vi "SR1.get Number of Lines.vi"(0 "i ref in":refnum<vi>, 5 "error in (no error)":errorcluster) -> (14 "i ref out":refnum<vi>, 16 "NofLines":i32, 19 "error out":errorcluster)   [LabVIEW 2014, in "SR1.lvlib"]
doc: "reads the number of FFT lines from the device"
uses:
  SR1.lvlib
  CSlibraries/UtilityLib/UtilityLib.valueStatus.ctl
  CS_Core/CSApplicationBaseClasses/NABase/NABase.directionType.ctl
  CS_Core/CSApplicationBaseClasses/NABase/NABase.serviceType.ctl
  CS_Core/CSSystem/CoreDefs/CoreDefs.error_type.ctl
  CS_Core/CSSystem/CoreLib/CoreLib.lvlib
  CSlibraries/UtilityLib/UtilityLib.lvlib
  CS_Core/CSApplicationBaseClasses/NABase/NABase.lvlib
  instr.lib/Stanford Research SR1/Stanford Research SR1.lvlib
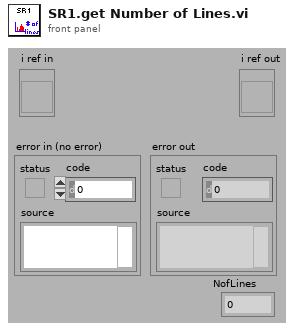
[diagram p1: front panel]
types:
  T1 = typedef "NABase.lvlib/NABase.serviceType.ctl" = enum16{"StartFreq", "NofLines", "FreqSpan", "status", "triggerLevel", "triggerSlope", "TimeRecDur", "NofStoredData"}
  T2 = typedef "NABase.lvlib/NABase.directionType.ctl" = enum16{"unknown", "update actual value", "update nominal value", "update both"}
  T3 = typedef "UtilityLib.lvlib/UtilityLib.valueStatus.ctl" = enum16{"no info available", "stand by/off", "on", "warning", "alarm/malfunction", "not implemented", "user action required", "important information", "system default", "control default", "indicator default", "button default"}
  T4 = typedef "CoreDefs.error_type.ctl" = enum16{"no error", "can't load process", "can't unload process", "process does not exist", "can't install process", "can't remove process", "unknown function", "time out", "can't execute function", "duplicate queue name", "super not found", "caller queue invalid", "can't ping process", "unknown error", "VISA Error", "VISA timeout", "GPIB timeout", "GPIB error", "communication error", "data type mismatch", "can't read data from OPC server", "can't write data to OPC server", "OET error", "function not implemented", "process already exists", "invalid Shared Variable name", "error writing Shared Variable", "error reading Shared Variable", "invalid client name", "corrupt database", "unknown class", "call not authorized", "parameter out of range", "OET timeout: can't get data to modify", "invalid queue name", "requested operation incompatible with current state", "event undefined", "event disabled", "state undefined", "caller is not a friend", "EventBuilder: bad eventID", "EventBuilder: no DAQ devices", "a thread must not stop itself", "UNUSED ELEMENT4", "DiscArchiver: eventData incomplete", "DiscArchiver: eventData does not belong to run", "DiscArchiver: can't open file", "DiscArchiver: can't write to file", "DiscArchiver: available disc space low", "can't acquire semaphore", "error reading data from database", "notifier object is not existing", "can't register process", "can't unregister process", "illegal event type", "object disabled", "object already exists", "can't change state", "Instrument not found", "no connection to remote node", "invalid reference", "N/A", "UNUSED ELEMENT 1", "element not found", "illegal TCP/IP connection detected", "object does not exist", "invalid access ID", "unknown CS system", "invalid privilige", "unsupported data type", "unsupported server type", "IO server already exists", "Shared Variable already exists"}
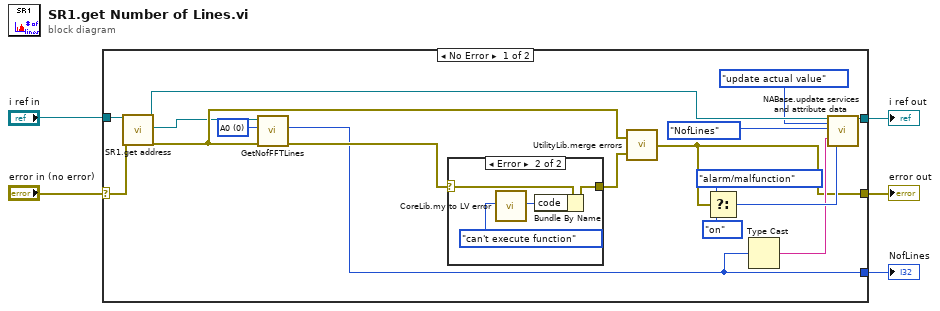
[diagram p0: block diagram]
diagram:
  n1 = case shown="No Error" "error in (no error)" {
    selector: "error in (no error)" -> [w20 w29]
    tunnel: "i ref in" -> [w22 w28]
    tunnel: [w13 w29] -> w4
    tunnel: [w14 w28] -> w3
    tunnel: [w6 _] -> w2
    frame No Error {
      w9 = 0 items=["A0", "A1"] ("Analyzer (0: A0)")
      n2 = call "SR1.get address.vi"("i ref in"=w22, "error in (no error)"=w20) -> ("i ref out"=w15:refnum<vi>, "VISA resource name"=w11:refnum<visa-resource-name>, "error out"=w12:errorcluster)  [unwired: 15 in]
      n3 = call "GetNofFFTLines.vi"("error in (no error)"=w12, "Analyzer (0: A0)"=w9, "VISA resource name"=w11) -> ("error out"=w10:errorcluster, "NofLines"=w6:i32)  [unwired: 6 in, 1 out]
      n4 = case shown="Error" w10 {
        selector: w10 -> [w23 w27]
        tunnel: [w23 w24] -> w21
        frame No Error {
        }
        frame Error {
          n5 = call "CoreLib.my to LV error.vi"("ErrorTypes"=CoreDefs.error_type."can't execute function") -> ("LV error code"=w26:i32)  [unwired: 17 in, 1 out]
          n6 = Bundle By Name(cluster=w27, "code"=w26) -> (w24:errorcluster)
        }
      }
      n7 = call "UtilityLib.merge errors.vi"("error2 (no error)"=w21, "error1 (no error)"=w12) -> ("error out"=w13:errorcluster)
      n8 = Select(t=UtilityLib.valueStatus."alarm/malfunction" ("quality"), s=w13, f=UtilityLib.valueStatus."on") -> (s? t:f=w17:T3)
      n9 = Type Cast(x=w6) -> (*(type *) &x=w16:string)  [unwired: 1 in]
      n10 = call "NABase.update services and attribute data.vi"("i ref in"=w15, "direction"=NABase.directionType."update actual value", "service"=NABase.serviceType."NofLines", "value"=w16, "quality"=w17) -> ("i ref out"=w14:refnum<vi>)  [unwired: 12 in, 2 out]
    }
    frame Error {
    }
  }
  "error out" <- w4
  "i ref out" <- w3
  "NofLines" <- w2
